vi "Write UPNC Enqueuer.vi"(8 "error in (no error)":errorcluster, 10 "Actor Framework.lvlib:Message Enqueuer":refnum<class "Message Enqueuer.lvclass">, 11 "UPNCalculatorGUI in":refnum<class "UPNCalculatorGUI.lvclass">) -> (0 "error out":errorcluster, 3 "UPNCalculatorGUI out":refnum<class "UPNCalculatorGUI.lvclass">)   [LabVIEW 2012, in "UPNCalculatorGUI Actor.lvlib" / "UPNCalculatorGUI.lvclass"]
uses:
  UPNCalculatorGUI.lvclass
  <vilib>/ActorFramework/Message Enqueuer/Message Enqueuer.lvclass
  UPNCalculatorGUI.lvclass/UPNCalculatorGUI.ctl
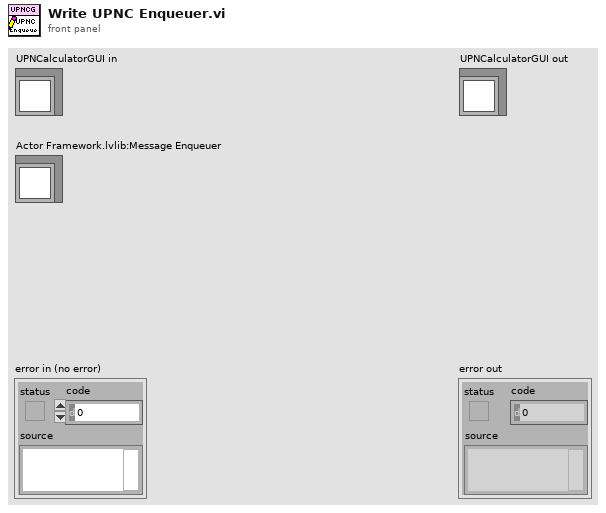
[diagram p1: front panel]
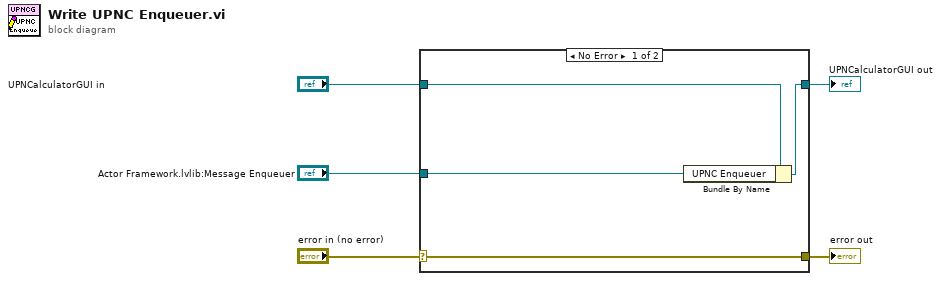
[diagram p0: block diagram]
diagram:
  n1 = case shown="No Error" "error in (no error)" {
    selector: "error in (no error)" -> [w9 w10]
    tunnel: [w9 w10] -> w4
    tunnel: [w7 w11] -> w2
    tunnel: "UPNCalculatorGUI in" -> [w8 w11]
    tunnel: "Actor Framework.lvlib:Message Enqueuer" -> [w6 _]
    frame No Error {
      n2 = Bundle By Name(cluster=w8, "UPNC Enqueuer"=w6) -> (w7:refnum<class "UPNCalculatorGUI.lvclass">)
    }
    frame Error {
    }
  }
  "error out" <- w4
  "UPNCalculatorGUI out" <- w2
